vi "Initialize Sentence.vi"(8 "error in":errorcluster, 11 "Sentence in":refnum<class "Sentence.lvclass">) -> (0 "error out":errorcluster, 3 "Sentence out":refnum<class "Sentence.lvclass">)   [LabVIEW 2016, in "Sentence.lvclass"]
uses:
  Sentence.lvclass
  C:/Users/Dzak/Documents/Projects/Evolutionary Programming/Genetic Algorithm Framework/IChromosome/IChromosome.lvclass
  Gene/Character.lvclass
  C:/Users/Dzak/Documents/Projects/Evolutionary Programming/Genetic Algorithm Framework/IGene/IGene.lvclass
  IChromosome/IChromosome.lvclass
panel:
  in  "# of Characters":u32=10
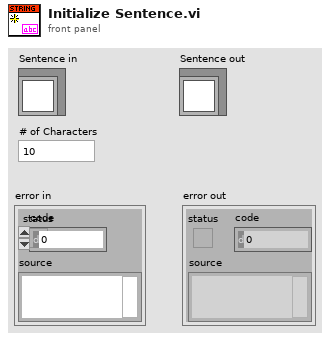
[diagram p1: front panel]
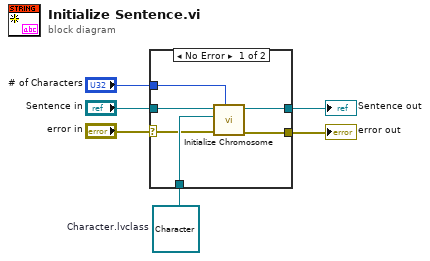
[diagram p0: block diagram]
diagram:
  w1 = refnum<class "Character.lvclass"> refnum  # Character.lvclass
  n1 = case shown="No Error" "error in" {
    selector: "error in" -> [w8 w14]
    tunnel: [w7 w14] -> w5
    tunnel: [w11 w13] -> w3
    tunnel: "Sentence in" -> [w12 w13]
    tunnel: "# of Characters" -> [w10 _]
    tunnel: w1 -> [w9 _]
    frame No Error {
      n2 = call "Initialize Chromosome.vi"("# of Genes"=w10, "error in"=w8, "Gene Type"=w9, "IChromosome in"=w12) -> ("error out"=w7:errorcluster, "IChromosome out"=w11:refnum<class "Sentence.lvclass">)  [unwired: 6 in]
    }
    frame Error {
    }
  }
  "error out" <- w5
  "Sentence out" <- w3
